vi "EOL CAN_Init CAL.vi"(5 "Parttype ref":refnum<vi>, 7 "Flash Size":i32, 8 "Glass?":bool=TRUE, 9 "Read Session in":refnum<k21>, 10 "DSC Write Session in":refnum<k21>, 11 "SA2 Operator":T1[](array[typedef]) {"Wert" format="%.0x"}) -> (1 "Error String Out":string, 2 "TxRx Data":string[][](array[string]), 3 "Response Good?":bool)   [LabVIEW 2014]
uses:
  Typedefs/Diagnose_SA2_Rechnenbefehl.ctl
  Typedefs/Diagnose_SA2_Operation_ENUM.ctl
  typedefs/parttype.ctl
  Typedefs/Select Session.ctl
  <vilib>/xnet/xnet.llb/XNET Frame CAN.ctl
  <vilib>/xnet/xnet.llb/XNET Frame Type CAN.ctl
panel:
  in  "Error String":string
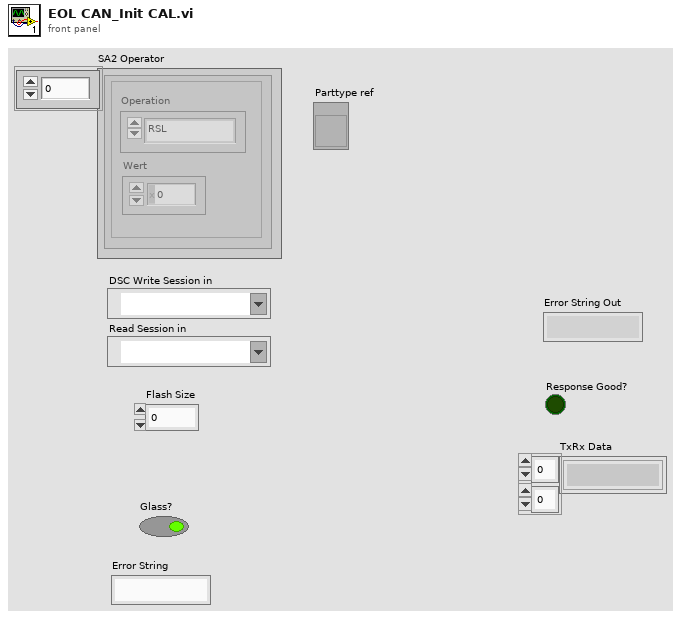
[diagram p1: front panel]
types:
  T1 = typedef "Diagnose_SA2_Rechnenbefehl.ctl" = cluster{"Operation":T2, "Wert":u32}
  T2 = typedef "Diagnose_SA2_Operation_ENUM.ctl" = enum16{"RSL", "RSR", "ADD", "SUB", "EOR", "Durchläufe", "NEXT", "BCC", "BRA", "Fertig"}
  T3 = cluster{"DSC Write Session in":refnum<k21>, "Read Session in":refnum<k21>, "Error String":string, "Response Good?":bool, "Glass?":bool, "TxRx Data":string[][], "SA2 Operator":T1[], "Flash Size":i32, "Parttype ref":refnum<vi>}
  T4 = typedef "Select Session.ctl" = enum16{"DefaultSession", "Development", "Extended", "EOL", "Programming"}
  T5 = typedef "XNET Frame CAN.ctl" = cluster{"timestamp":timestamp, "payload":u8[], "identifier":u32, "type":T6, "extended?":bool, "echo?":bool}
  T6 = typedef "XNET Frame Type CAN.ctl" = u8
  T7 = typedef "parttype.ctl" = enum16{"NMS", "B-SUV"}
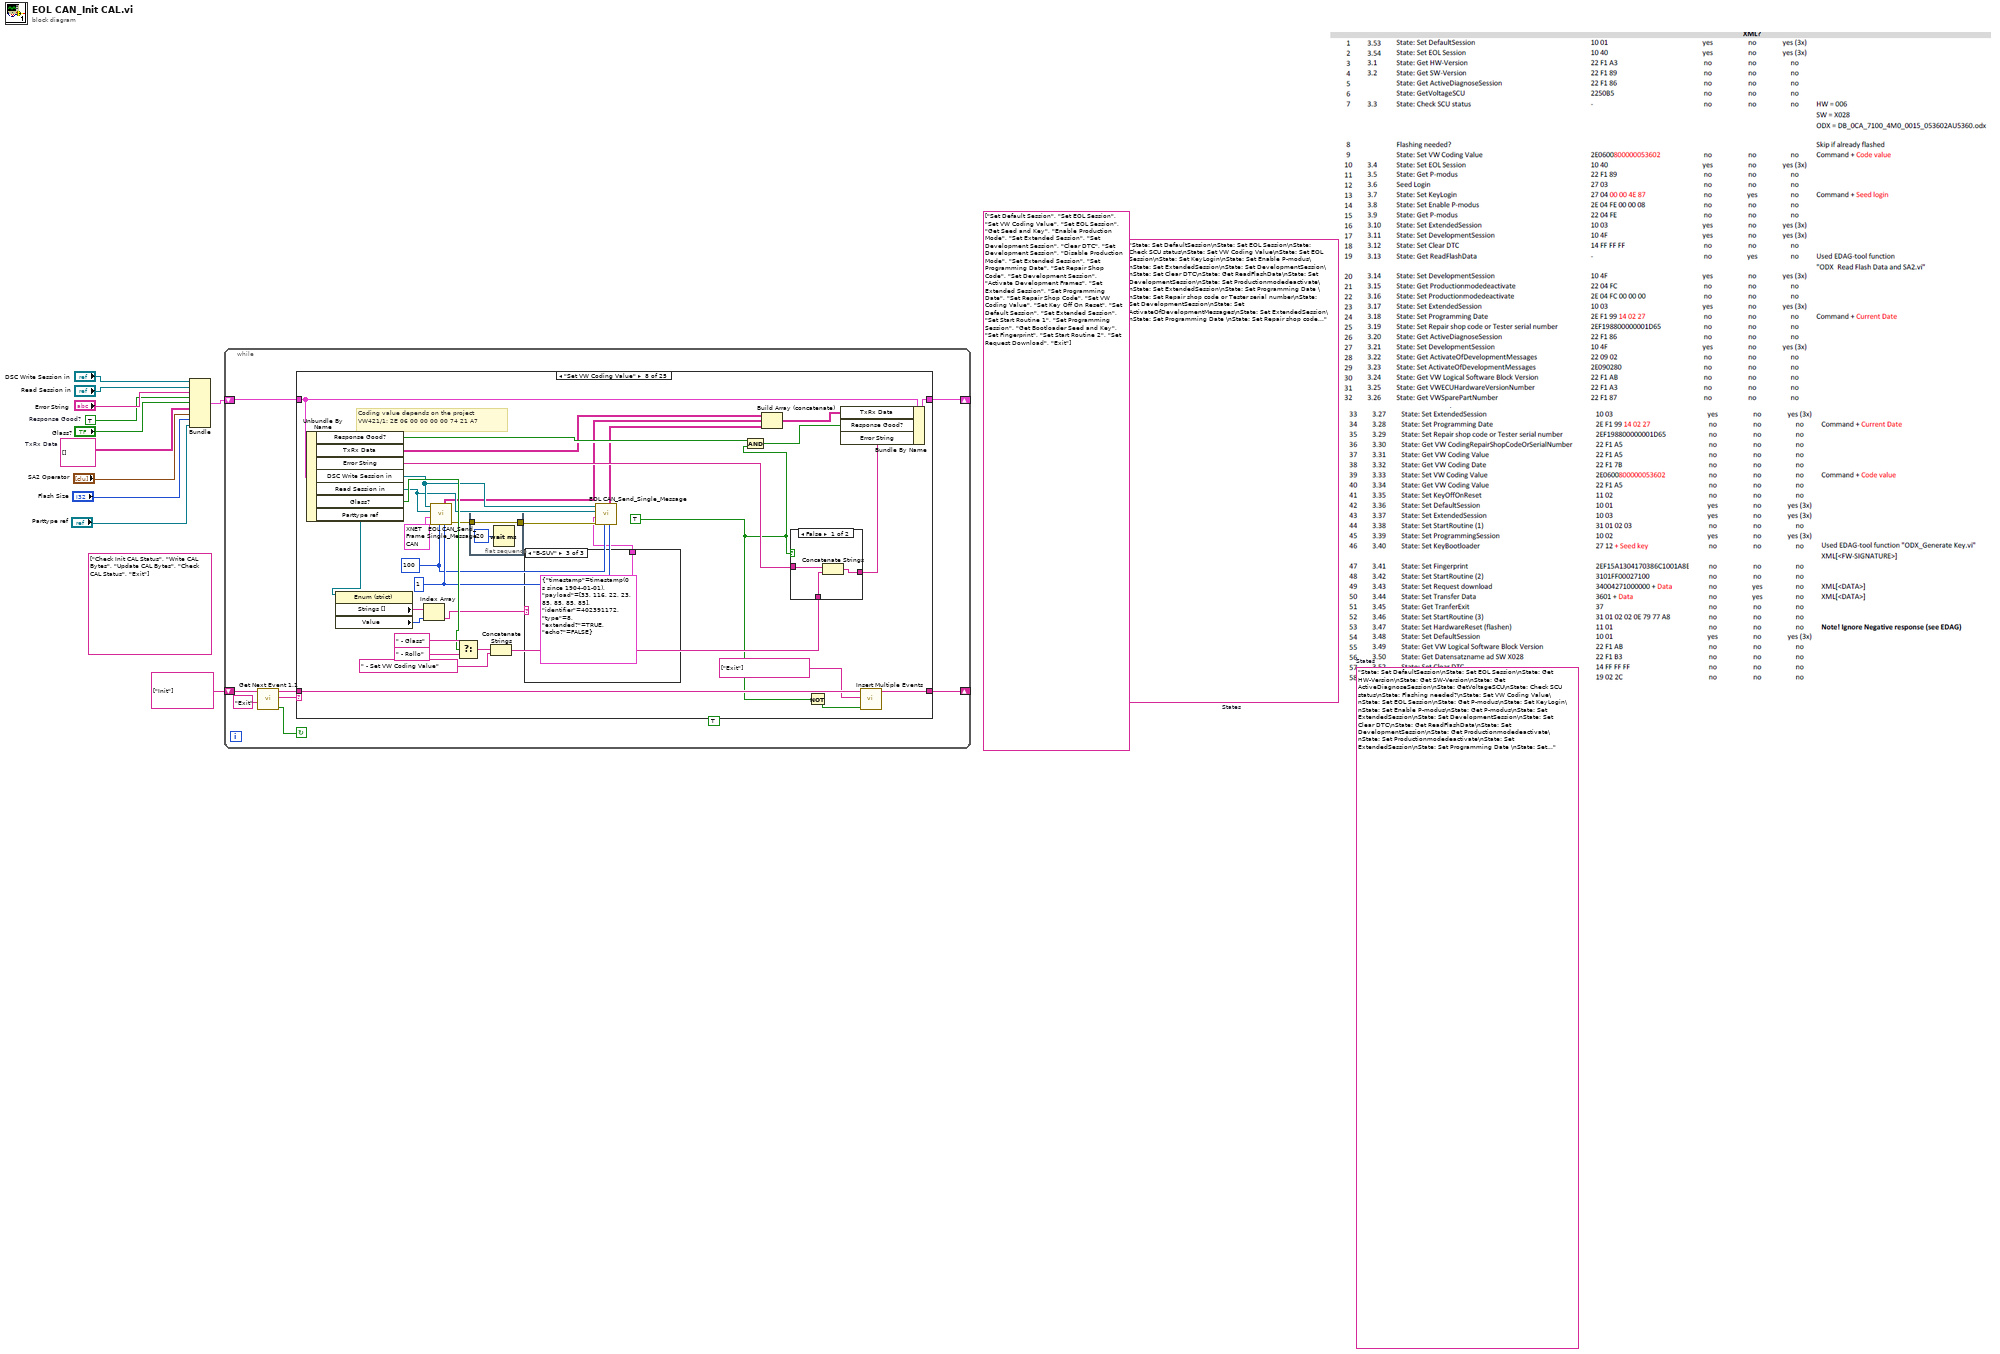
[diagram p0: block diagram]
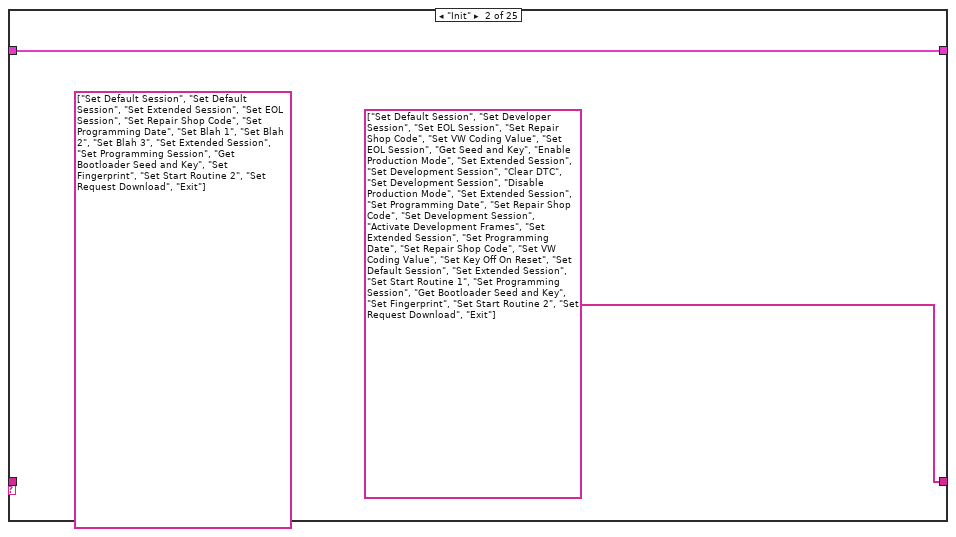
[diagram p3: hidden frame]
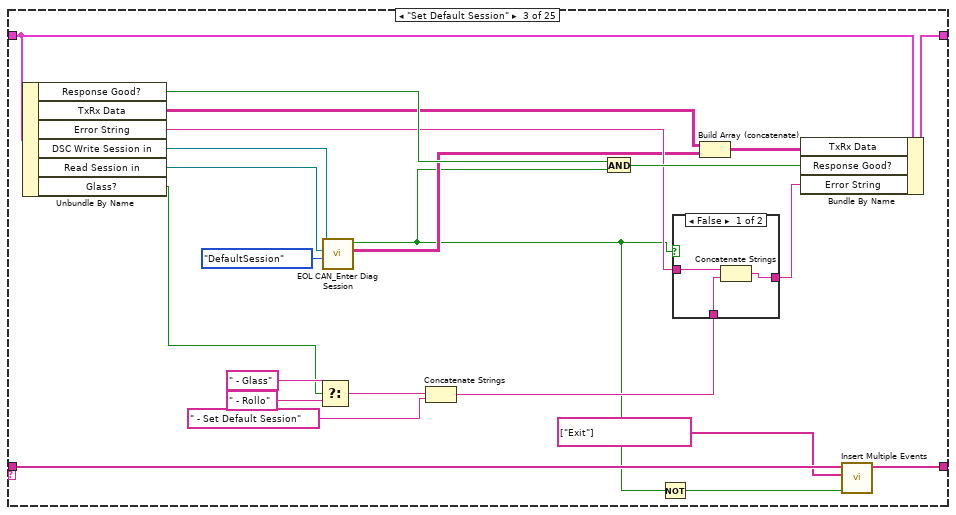
[diagram p4: hidden frame]
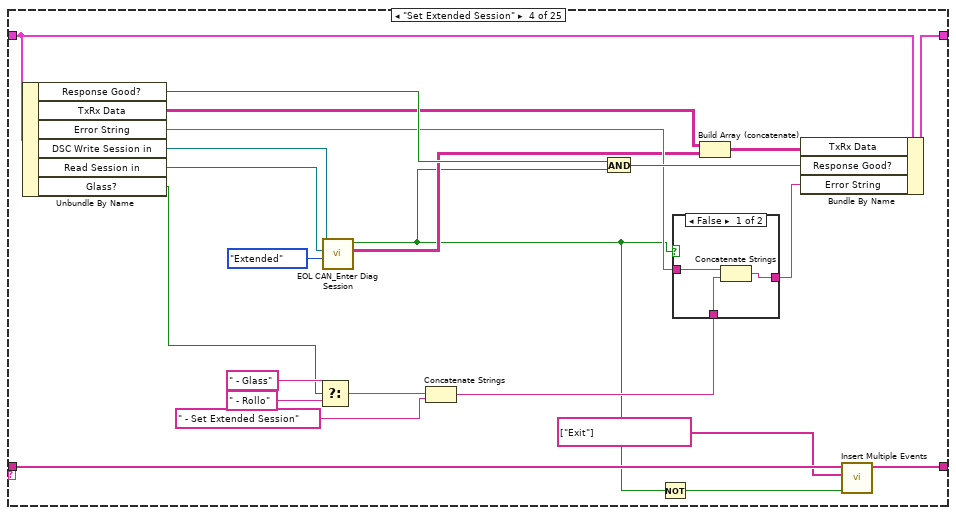
[diagram p6: hidden frame]
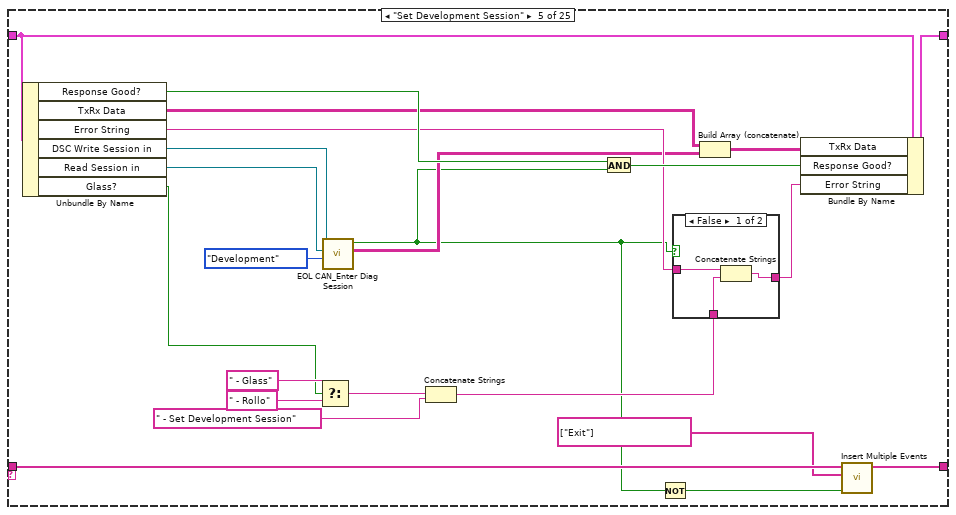
[diagram p8: hidden frame]
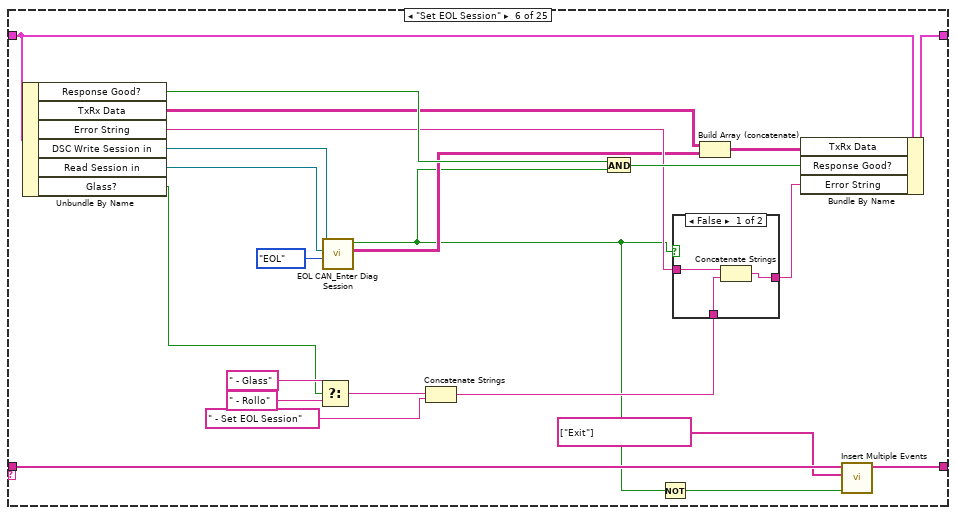
[diagram p10: hidden frame]
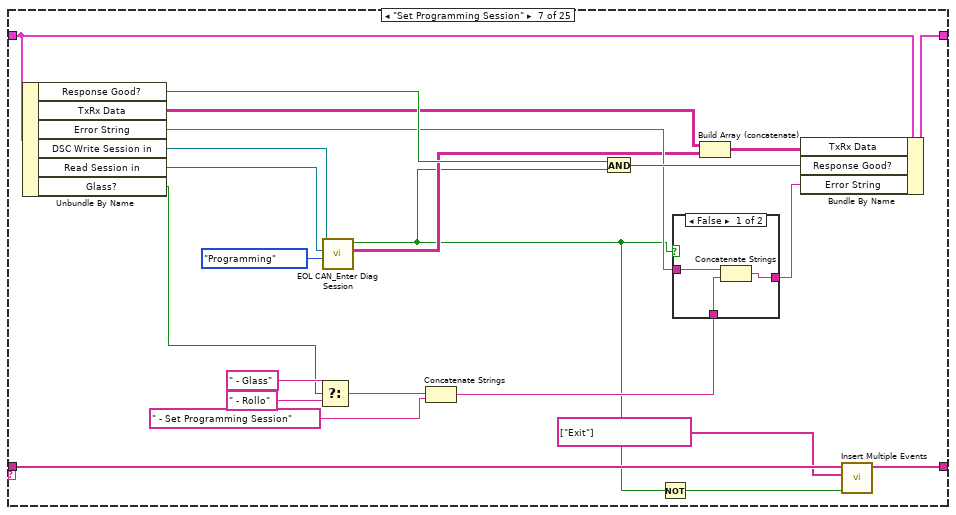
[diagram p12: hidden frame]
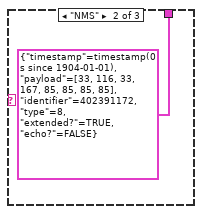
[diagram p15: hidden frame]
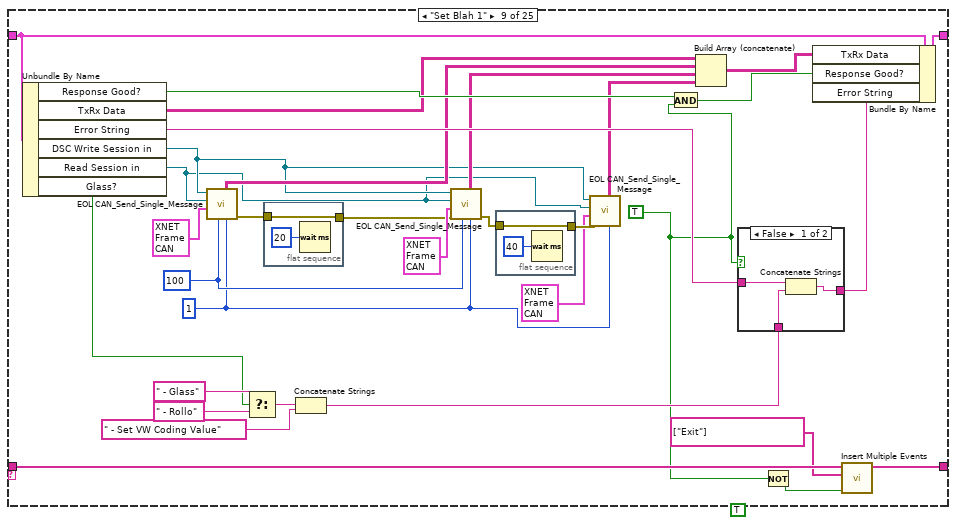
[diagram p17: hidden frame]
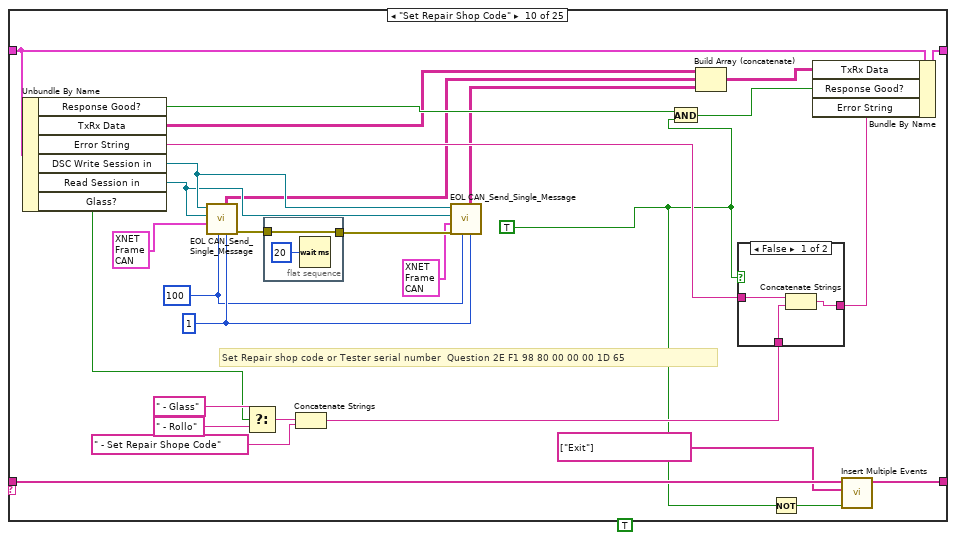
[diagram p19: hidden frame]
diagram:
  (unwired) "State: Set DefaultSession\nState: Set EOL Session\nState: Get HW-Version\nState: Get SW-Version\nState: Get ActiveDiagnoseSession\nState: GetVoltageSCU\nState: Check SCU status\nState: Flashing needed?\nState: Set VW Coding Value\nState: Set EOL Session\nState: Get P-modus\nState: Set KeyLogin\nState: Set Enable P-modus\nState: Get P-modus\nState: Set ExtendedSession\nState: Set DevelopmentSession\nState: Set Clear DTC\nState: Get ReadFlashData\nState: Set DevelopmentSession\nState: Get Productionmodedeactivate\nState: Set Productionmodedeactivate\nState: Set ExtendedSession\nState: Set Programming Date \nState: Set Repair shop code or Tester serial number\nState: Get ActiveDiagnoseSession \nState: Set DevelopmentSession\nState: Get ActivateOfDevelopmentMessages\nState: Set ActivateOfDevelopmentMessages\nState: Get VW Logical Software Block Version\nState: Get VWECUHardwareVersionNumber\nState: Get VWSparePartNumber\nState: Set ExtendedSession\nState: Set Programming Date \nState: Set Repair shop code or Tester serial number\nState: Get VW CodingRepairShopCodeOrSerialNumber\nState: Get VW Coding Value\nState: Get VW Coding Date\nState: Set VW Coding Value\nState: Get VW Coding Value\nState: Set KeyOffOnReset\nState: Set DefaultSession\nState: Set ExtendedSession\nState: Set StartRoutine (1)\nState: Set ProgrammingSession\nState: Set KeyBootloader\nState: Set Fingerprint\nState: Set StartRoutine (2)\nState: Set Request download\nState: Set Transfer Data\nState: Get TranferExit\nState: Set StartRoutine (3)\nState: Get ActiveDiagnoseSession \nState: Set HardwareReset (flashen)\nState: Set DefaultSession\nState: Get VW Logical Software Block Version\nState: Get Datensatzname ad SW X028\nState: Set Clear DTC\nState: Get DTC (TestFailed + Confirmed DTC)\nExit"  # States
  (unwired) "State: Set DefaultSession\nState: Set EOL Session\nState: Check SCU status\nState: Set VW Coding Value\nState: Set EOL Session\nState: Set KeyLogin\nState: Set Enable P-modus\nState: Set ExtendedSession\nState: Set DevelopmentSession\nState: Set Clear DTC\nState: Get ReadFlashData\nState: Set DevelopmentSession\nState: Set Productionmodedeactivate\nState: Set ExtendedSession\nState: Set Programming Date \nState: Set Repair shop code or Tester serial number\nState: Set DevelopmentSession\nState: Set ActivateOfDevelopmentMessages\nState: Set ExtendedSession\nState: Set Programming Date \nState: Set Repair shop code or Tester serial number\nState: Set VW Coding Value\nState: Set KeyOffOnReset\nState: Set DefaultSession\nState: Set ExtendedSession\nState: Set StartRoutine (1)\nState: Set ProgrammingSession\nState: Set KeyBootloader\nState: Set Fingerprint\nState: Set StartRoutine (2)\nState: Set Request download\nState: Set Transfer Data\nState: Get TranferExit\nState: Set StartRoutine (3)\nState: Set HardwareReset (flashen)\nState: Set DefaultSession\nState: Get Datensatzname ad SW X028\nState: Set Clear DTC\nState: Get DTC (TestFailed + Confirmed DTC)\nExit"  # States
  (unwired) string[] ["Set Default Session", "Set EOL Session", "Set VW Coding Value", "Set EOL Session", "Get Seed and Key", "Enable Production Mode", "Set Extended Session", "Set Development Session", "Clear DTC", "Set Development Session", "Disable Production Mode", "Set Extended Session", "Set Programming Date", "Set Repair Shop Code", "Set Development Session", "Activate Development Frames", "Set Extended Session", "Set Programming Date", "Set Repair Shop Code", "Set VW Coding Value", "Set Key Off On Reset", "Set Default Session", "Set Extended Session", "Set Start Routine 1", "Set Programming Session", "Get Bootloader Seed and Key", "Set Fingerprint", "Set Start Routine 2", "Set Request Download", "Exit"] ("event queue out")
  (unwired) string[] ["Check Init CAL Status", "Write CAL Bytes", "Update CAL Bytes", "Check CAL Status", "Exit"] ("event queue out")
  w6 = string[][] []  # TxRx Data
  w9 = TRUE  # Response Good?
  n1 = Bundle("DSC Write Session in"="DSC Write Session in", "Read Session in"="Read Session in", "Error String"="Error String", "Response Good?"=w9, "Glass?"="Glass?", "TxRx Data"=w6, "SA2 Operator"="SA2 Operator", "Flash Size"="Flash Size", "Parttype ref"="Parttype ref") -> (w8:T3)  [unwired: 1 in]
  n2 = while {
    shift-right: [w17] -> _
    shift-left: string[] ["Init"] ("event queue out") -> [w16]
    shift-right: [w14] -> _
    shift-left: w8 -> [w15]
    stop <- w19 continue-if-true
    n3 = call "Get Next Event 1.1.vi"("Exit Event"="Exit", "event queue in"=w16) -> ("Condition (Exit:F)"=w19:bool, "next event"=w12:string, "event queue out"=w18:string[])  [unwired: 6 in, 1 out]
    n4 = case shown="\"Set VW Coding Value\"" w12 {
      tunnel: w18 -> [w21 _ w34 w61 w88 w115 w142 w179 w220 w257 w298 w333 w361 w388 w414 w440 w477 w507 w538 w567 w594 w621 w648 w674 w695]
      tunnel: [w21 string[] ["Set Default Session", "Set Developer Session", "Set EOL Session", "Set Repair Shop Code", "Set VW Coding Value", "Set EOL Session", "Get Seed and Key", "Enable Production Mode", "Set Extended Session", "Set Development Session", "Clear DTC", "Set Development Session", "Disable Production Mode", "Set Extended Session", "Set Programming Date", "Set Repair Shop Code", "Set Development Session", "Activate Development Frames", "Set Extended Session", "Set Programming Date", "Set Repair Shop Code", "Set VW Coding Value", "Set Key Off On Reset", "Set Default Session", "Set Extended Session", "Set Start Routine 1", "Set Programming Session", "Get Bootloader Seed and Key", "Set Fingerprint", "Set Start Routine 2", "Set Request Download", "Exit"] ("event queue out") w35 w62 w89 w116 w143 w180 w221 w258 w299 w334 w362 w389 w415 w441 w478 w508 w539 w568 w595 w622 w649 w675 w695] -> w17
      tunnel: w15 -> [w20 w23 w45 w72 w99 w126 w153 w190 w231 w268 w309 w344 w372 w399 w425 w451 w488 w518 w549 w578 w605 w632 w659 w685 w694]
      tunnel: [w20 w23 w43 w70 w97 w124 w151 w188 w229 w266 w307 w342 w370 w397 w423 w449 w486 w516 w547 w576 w603 w630 w657 w683 w694] -> w14
      frame "Error", Default {
      }
      frame "Init" {
        (unwired) string[] ["Set Default Session", "Set Default Session", "Set Extended Session", "Set EOL Session", "Set Repair Shop Code", "Set Programming Date", "Set Blah 1", "Set Blah 2", "Set Blah 3", "Set Extended Session", "Set Programming Session", "Get Bootloader Seed and Key", "Set Fingerprint", "Set Start Routine 2", "Set Request Download", "Exit"] ("event queue out")
        # "Inalfa Sequences"
        # "Conti-Sequences"
      }
      frame "Set Default Session" {
        n5 = Unbundle By Name(w45) -> ("Response Good?"=w46:bool, "TxRx Data"=w32:string[][], "Error String"=w42:string, "DSC Write Session in"=w29:refnum<k21>, "Read Session in"=w28:refnum<k21>, "Glass?"=w26:bool)
        n6 = Select(t=" - Glass" ("Error Description"), s=w26, f=" - Rollo" ("Error Description")) -> (s? t:f=w40:string)
        n7 = call "EOL CAN_Enter Diag Session.vi"("Session"=Select_Session."DefaultSession", "Read Session in"=w28, "Write Session in"=w29) -> ("TxRx Data"=w30:string[][], "Response Good?"=w25:bool)  [unwired: 6 in, 1 out]
        n8 = Concatenate Strings(w40, " - Set Default Session" ("Error Description")) -> (w36:string)
        n9 = And(x=w46, y=w25) -> (x .and. y?=w44:bool)
        n10 = Not(x=w25) -> (.not. x?=w24:bool)
        n11 = case shown="False" w25 {
          tunnel: w42 -> [w48 w50]
          tunnel: [w49 w50] -> w41
          tunnel: w36 -> [w47 _]
          frame False {
            n12 = Concatenate Strings(w48, w47) -> (w49:string)
          }
          frame True {
          }
        }
        n13 = Build Array (concatenate)(w32, w30) -> (w31:string[][])
        n14 = Bundle By Name(cluster=w45, "TxRx Data"=w31, "Response Good?"=w44, "Error String"=w41) -> (w43:T3)
        n15 = call "Insert Multiple Events.vi"("Insert all? (T)"=w24, "Events to Insert"=string[] ["Exit"], "Event queue in"=w34) -> ("Event queue out"=w35:string[])  [unwired: 4 in]
      }
      frame "Set Extended Session" {
        n16 = Unbundle By Name(w72) -> ("Response Good?"=w73:bool, "TxRx Data"=w59:string[][], "Error String"=w69:string, "DSC Write Session in"=w56:refnum<k21>, "Read Session in"=w55:refnum<k21>, "Glass?"=w53:bool)
        n17 = Select(t=" - Glass" ("Error Description"), s=w53, f=" - Rollo" ("Error Description")) -> (s? t:f=w67:string)
        n18 = call "EOL CAN_Enter Diag Session.vi"("Session"=Select_Session."Extended", "Read Session in"=w55, "Write Session in"=w56) -> ("TxRx Data"=w57:string[][], "Response Good?"=w52:bool)  [unwired: 6 in, 1 out]
        n19 = Concatenate Strings(w67, " - Set Extended Session" ("Error Description")) -> (w63:string)
        n20 = And(x=w73, y=w52) -> (x .and. y?=w71:bool)
        n21 = Not(x=w52) -> (.not. x?=w51:bool)
        n22 = case shown="False" w52 {
          tunnel: w69 -> [w75 w77]
          tunnel: [w76 w77] -> w68
          tunnel: w63 -> [w74 _]
          frame False {
            n23 = Concatenate Strings(w75, w74) -> (w76:string)
          }
          frame True {
          }
        }
        n24 = Build Array (concatenate)(w59, w57) -> (w58:string[][])
        n25 = Bundle By Name(cluster=w72, "TxRx Data"=w58, "Response Good?"=w71, "Error String"=w68) -> (w70:T3)
        n26 = call "Insert Multiple Events.vi"("Insert all? (T)"=w51, "Events to Insert"=string[] ["Exit"], "Event queue in"=w61) -> ("Event queue out"=w62:string[])  [unwired: 4 in]
      }
      frame "Set Development Session" {
        n27 = Unbundle By Name(w99) -> ("Response Good?"=w100:bool, "TxRx Data"=w86:string[][], "Error String"=w96:string, "DSC Write Session in"=w83:refnum<k21>, "Read Session in"=w82:refnum<k21>, "Glass?"=w80:bool)
        n28 = Select(t=" - Glass" ("Error Description"), s=w80, f=" - Rollo" ("Error Description")) -> (s? t:f=w94:string)
        n29 = call "EOL CAN_Enter Diag Session.vi"("Session"=Select_Session."Development", "Read Session in"=w82, "Write Session in"=w83) -> ("TxRx Data"=w84:string[][], "Response Good?"=w79:bool)  [unwired: 6 in, 1 out]
        n30 = Concatenate Strings(w94, " - Set Development Session" ("Error Description")) -> (w90:string)
        n31 = And(x=w100, y=w79) -> (x .and. y?=w98:bool)
        n32 = Not(x=w79) -> (.not. x?=w78:bool)
        n33 = case shown="False" w79 {
          tunnel: w96 -> [w102 w104]
          tunnel: [w103 w104] -> w95
          tunnel: w90 -> [w101 _]
          frame False {
            n34 = Concatenate Strings(w102, w101) -> (w103:string)
          }
          frame True {
          }
        }
        n35 = Build Array (concatenate)(w86, w84) -> (w85:string[][])
        n36 = Bundle By Name(cluster=w99, "TxRx Data"=w85, "Response Good?"=w98, "Error String"=w95) -> (w97:T3)
        n37 = call "Insert Multiple Events.vi"("Insert all? (T)"=w78, "Events to Insert"=string[] ["Exit"], "Event queue in"=w88) -> ("Event queue out"=w89:string[])  [unwired: 4 in]
      }
      frame "Set EOL Session" {
        n38 = Unbundle By Name(w126) -> ("Response Good?"=w127:bool, "TxRx Data"=w113:string[][], "Error String"=w123:string, "DSC Write Session in"=w110:refnum<k21>, "Read Session in"=w109:refnum<k21>, "Glass?"=w107:bool)
        n39 = Select(t=" - Glass" ("Error Description"), s=w107, f=" - Rollo" ("Error Description")) -> (s? t:f=w121:string)
        n40 = call "EOL CAN_Enter Diag Session.vi"("Session"=Select_Session."EOL", "Read Session in"=w109, "Write Session in"=w110) -> ("TxRx Data"=w111:string[][], "Response Good?"=w106:bool)  [unwired: 6 in, 1 out]
        n41 = Concatenate Strings(w121, " - Set EOL Session" ("Error Description")) -> (w117:string)
        n42 = And(x=w127, y=w106) -> (x .and. y?=w125:bool)
        n43 = Not(x=w106) -> (.not. x?=w105:bool)
        n44 = case shown="False" w106 {
          tunnel: w123 -> [w129 w131]
          tunnel: [w130 w131] -> w122
          tunnel: w117 -> [w128 _]
          frame False {
            n45 = Concatenate Strings(w129, w128) -> (w130:string)
          }
          frame True {
          }
        }
        n46 = Build Array (concatenate)(w113, w111) -> (w112:string[][])
        n47 = Bundle By Name(cluster=w126, "TxRx Data"=w112, "Response Good?"=w125, "Error String"=w122) -> (w124:T3)
        n48 = call "Insert Multiple Events.vi"("Insert all? (T)"=w105, "Events to Insert"=string[] ["Exit"], "Event queue in"=w115) -> ("Event queue out"=w116:string[])  [unwired: 4 in]
      }
      frame "Set Programming Session" {
        n49 = Unbundle By Name(w153) -> ("Response Good?"=w154:bool, "TxRx Data"=w140:string[][], "Error String"=w150:string, "DSC Write Session in"=w137:refnum<k21>, "Read Session in"=w136:refnum<k21>, "Glass?"=w134:bool)
        n50 = Select(t=" - Glass" ("Error Description"), s=w134, f=" - Rollo" ("Error Description")) -> (s? t:f=w148:string)
        n51 = call "EOL CAN_Enter Diag Session.vi"("Session"=Select_Session."Programming", "Read Session in"=w136, "Write Session in"=w137) -> ("TxRx Data"=w138:string[][], "Response Good?"=w133:bool)  [unwired: 6 in, 1 out]
        n52 = Concatenate Strings(w148, " - Set Programming Session" ("Error Description")) -> (w144:string)
        n53 = And(x=w154, y=w133) -> (x .and. y?=w152:bool)
        n54 = Not(x=w133) -> (.not. x?=w132:bool)
        n55 = case shown="False" w133 {
          tunnel: w150 -> [w156 w158]
          tunnel: [w157 w158] -> w149
          tunnel: w144 -> [w155 _]
          frame False {
            n56 = Concatenate Strings(w156, w155) -> (w157:string)
          }
          frame True {
          }
        }
        n57 = Build Array (concatenate)(w140, w138) -> (w139:string[][])
        n58 = Bundle By Name(cluster=w153, "TxRx Data"=w139, "Response Good?"=w152, "Error String"=w149) -> (w151:T3)
        n59 = call "Insert Multiple Events.vi"("Insert all? (T)"=w132, "Events to Insert"=string[] ["Exit"], "Event queue in"=w142) -> ("Event queue out"=w143:string[])  [unwired: 4 in]
      }
      frame "Set VW Coding Value" {
        w164 = TRUE ("Response Good?")
        (unwired) TRUE ("Insert all? (T)")
        w171 = 1 ("Retries")
        w170 = u32 100 ("Msg Wait Time")
        # "Coding value depends on the project\nVW421/1: 2E 06 00 00 00 00 74 21 A7"
        n60 = Unbundle By Name(w190) -> ("Response Good?"=w191:bool, "TxRx Data"=w177:string[][], "Error String"=w187:string, "DSC Write Session in"=w173:refnum<k21>, "Read Session in"=w172:refnum<k21>, "Glass?"=w175:bool, "Parttype ref"=w160:refnum<vi>)
        n61 = property class="Enum (strict)"(reference=w160) -> ("Strings []"=w161:string[], "Value"=w162:T7)  [unwired: 1 in, 2 out]
        n62 = Index Array(array=w161, index=w162) -> (element=w159:string)
        n63 = call "EOL CAN_Send_Single_Message.vi"("Retries"=w171, "Msg Wait Time"=w170, "Tx CAN frame"=T5 {"timestamp"=timestamp(0 s since 1904-01-01), "payload"=[16, 9, 46, 6, 0, 0, 0, 0], "identifier"=402391172, "type"=8, "extended?"=TRUE, "echo?"=FALSE}, "Read Session in"=w172, "Write Session in"=w173) -> ("Error out"=w167:errorcluster, "TxRx Data"=w169:string[][])  [unwired: 2 in, 3 out]
        n64 = Select(t=" - Glass" ("Error Description"), s=w175, f=" - Rollo" ("Error Description")) -> (s? t:f=w185:string)
        n65 = flat-sequence {
          tunnel: w167 -> [w195]
          tunnel: [w195] -> w166
          frame #0 {
            n66 = Wait (ms)(milliseconds to wait=u32 20) -> ()  [unwired: 1 out]
          }
        }
        n67 = Concatenate Strings(w185, " - Set VW Coding Value" ("Error Description")) -> (w181:string)
        n68 = case shown="\"B-SUV\"" w159 {
          tunnel: [_ T5 {"timestamp"=timestamp(0 s since 1904-01-01), "payload"=[33, 116, 33, 167, 85, 85, 85, 85], "identifier"=402391172, "type"=8, "extended?"=TRUE, "echo?"=FALSE} ("Tx CAN frame") T5 {"timestamp"=timestamp(0 s since 1904-01-01), "payload"=[33, 116, 22, 23, 85, 85, 85, 85], "identifier"=402391172, "type"=8, "extended?"=TRUE, "echo?"=FALSE} ("Tx CAN frame")] -> w163
          frame "NaN", Default {
          }
          frame "NMS" {
          }
          frame "B-SUV" {
          }
        }
        n69 = call "EOL CAN_Send_Single_Message.vi"("Retries"=w171, "Msg Wait Time"=w170, "Error in"=w166, "Tx CAN frame"=w163, "Read Session in"=w172, "Write Session in"=w173) -> ("TxRx Data"=w168:string[][])  [unwired: 1 in, 4 out]
        n70 = And(x=w191, y=w164) -> (x .and. y?=w189:bool)
        n71 = Build Array (concatenate)(w177, w169, w168) -> (w176:string[][])
        n72 = case shown="False" w164 {
          tunnel: w187 -> [w197 w199]
          tunnel: [w198 w199] -> w186
          tunnel: w181 -> [w196 _]
          frame False {
            n73 = Concatenate Strings(w197, w196) -> (w198:string)
          }
          frame True {
          }
        }
        n74 = Not(x=w164) -> (.not. x?=w165:bool)
        n75 = Bundle By Name(cluster=w190, "TxRx Data"=w176, "Response Good?"=w189, "Error String"=w186) -> (w188:T3)
        n76 = call "Insert Multiple Events.vi"("Insert all? (T)"=w165, "Events to Insert"=string[] ["Exit"], "Event queue in"=w179) -> ("Event queue out"=w180:string[])  [unwired: 4 in]
      }
      frame "Set Blah 1" {
        w207 = TRUE ("Response Good?")
        (unwired) TRUE ("Insert all? (T)")
        w200 = 1 ("Retries")
        w213 = u32 100 ("Msg Wait Time")
        n77 = Unbundle By Name(w231) -> ("Response Good?"=w232:bool, "TxRx Data"=w218:string[][], "Error String"=w228:string, "DSC Write Session in"=w204:refnum<k21>, "Read Session in"=w203:refnum<k21>, "Glass?"=w216:bool)
        n78 = call "EOL CAN_Send_Single_Message.vi"("Retries"=w200, "Msg Wait Time"=w213, "Tx CAN frame"=T5 {"timestamp"=timestamp(0 s since 1904-01-01), "payload"=[16, 14, 46, 241, 160, 67, 111, 110], "identifier"=402391172, "type"=8, "extended?"=TRUE, "echo?"=FALSE}, "Read Session in"=w203, "Write Session in"=w204) -> ("Error out"=w210:errorcluster, "TxRx Data"=w212:string[][])  [unwired: 2 in, 3 out]
        n79 = Select(t=" - Glass" ("Error Description"), s=w216, f=" - Rollo" ("Error Description")) -> (s? t:f=w226:string)
        n80 = flat-sequence {
          tunnel: w210 -> [w236]
          tunnel: [w236] -> w209
          frame #0 {
            n81 = Wait (ms)(milliseconds to wait=u32 20) -> ()  [unwired: 1 out]
          }
        }
        n82 = Concatenate Strings(w226, " - Set VW Coding Value" ("Error Description")) -> (w222:string)
        n83 = call "EOL CAN_Send_Single_Message.vi"("Retries"=w200, "Msg Wait Time"=w213, "Error in"=w209, "Tx CAN frame"=T5 {"timestamp"=timestamp(0 s since 1904-01-01), "payload"=[33, 116, 105, 110, 101, 110, 116, 97], "identifier"=402391172, "type"=8, "extended?"=TRUE, "echo?"=FALSE}, "Read Session in"=w203, "Write Session in"=w204) -> ("Error out"=w206:errorcluster, "TxRx Data"=w211:string[][])  [unwired: 1 in, 3 out]
        n84 = flat-sequence {
          tunnel: w206 -> [w234]
          tunnel: [w234] -> w205
          frame #0 {
            n85 = Wait (ms)(milliseconds to wait=u32 40) -> ()  [unwired: 1 out]
          }
        }
        n86 = call "EOL CAN_Send_Single_Message.vi"("Retries"=w200, "Error in"=w205, "Tx CAN frame"=T5 {"timestamp"=timestamp(0 s since 1904-01-01), "payload"=[34, 108, 85, 85, 85, 85, 85, 85], "identifier"=402391172, "type"=8, "extended?"=TRUE, "echo?"=FALSE}, "Read Session in"=w203, "Write Session in"=w204) -> ("TxRx Data"=w201:string[][])  [unwired: 2 in, 4 out]
        n87 = And(x=w232, y=w207) -> (x .and. y?=w230:bool)
        n88 = Build Array (concatenate)(w218, w212, w211, w201) -> (w217:string[][])
        n89 = case shown="False" w207 {
          tunnel: w228 -> [w238 w240]
          tunnel: [w239 w240] -> w227
          tunnel: w222 -> [w237 _]
          frame False {
            n90 = Concatenate Strings(w238, w237) -> (w239:string)
          }
          frame True {
          }
        }
        n91 = Not(x=w207) -> (.not. x?=w208:bool)
        n92 = Bundle By Name(cluster=w231, "TxRx Data"=w217, "Response Good?"=w230, "Error String"=w227) -> (w229:T3)
        n93 = call "Insert Multiple Events.vi"("Insert all? (T)"=w208, "Events to Insert"=string[] ["Exit"], "Event queue in"=w220) -> ("Event queue out"=w221:string[])  [unwired: 4 in]
      }
      frame "Set Repair Shop Code" {
        w243 = TRUE ("Response Good?")
        (unwired) TRUE ("Insert all? (T)")
        w250 = 1 ("Retries")
        w249 = u32 100 ("Msg Wait Time")
        # "Set Repair shop code or Tester serial number \tQuestion\t2E F1 98 80 00 00 00 1D 65"
        n94 = Unbundle By Name(w268) -> ("Response Good?"=w269:bool, "TxRx Data"=w255:string[][], "Error String"=w265:string, "DSC Write Session in"=w252:refnum<k21>, "Read Session in"=w251:refnum<k21>, "Glass?"=w253:bool)
        n95 = call "EOL CAN_Send_Single_Message.vi"("Retries"=w250, "Msg Wait Time"=w249, "Tx CAN frame"=T5 {"timestamp"=timestamp(0 s since 1904-01-01), "payload"=[16, 9, 46, 241, 152, 128, 0, 0], "identifier"=402391172, "type"=8, "extended?"=TRUE, "echo?"=FALSE}, "Read Session in"=w251, "Write Session in"=w252) -> ("Error out"=w246:errorcluster, "TxRx Data"=w248:string[][])  [unwired: 2 in, 3 out]
        n96 = Select(t=" - Glass" ("Error Description"), s=w253, f=" - Rollo" ("Error Description")) -> (s? t:f=w263:string)
        n97 = flat-sequence {
          tunnel: w246 -> [w271]
          tunnel: [w271] -> w245
          frame #0 {
            n98 = Wait (ms)(milliseconds to wait=u32 20) -> ()  [unwired: 1 out]
          }
        }
        n99 = Concatenate Strings(w263, " - Set Repair Shope Code" ("Error Description")) -> (w259:string)
        n100 = call "EOL CAN_Send_Single_Message.vi"("Retries"=w250, "Msg Wait Time"=w249, "Error in"=w245, "Tx CAN frame"=T5 {"timestamp"=timestamp(0 s since 1904-01-01), "payload"=[33, 0, 29, 101, 85, 85, 85, 85], "identifier"=402391172, "type"=8, "extended?"=TRUE, "echo?"=FALSE}, "Read Session in"=w251, "Write Session in"=w252) -> ("TxRx Data"=w247:string[][])  [unwired: 1 in, 4 out]
        n101 = And(x=w269, y=w243) -> (x .and. y?=w267:bool)
        n102 = Build Array (concatenate)(w255, w248, w247) -> (w254:string[][])
        n103 = case shown="False" w243 {
          tunnel: w265 -> [w273 w275]
          tunnel: [w274 w275] -> w264
          tunnel: w259 -> [w272 _]
          frame False {
            n104 = Concatenate Strings(w273, w272) -> (w274:string)
          }
          frame True {
          }
        }
        n105 = Not(x=w243) -> (.not. x?=w244:bool)
        n106 = Bundle By Name(cluster=w268, "TxRx Data"=w254, "Response Good?"=w267, "Error String"=w264) -> (w266:T3)
        n107 = call "Insert Multiple Events.vi"("Insert all? (T)"=w244, "Events to Insert"=string[] ["Exit"], "Event queue in"=w257) -> ("Event queue out"=w258:string[])  [unwired: 4 in]
      }
      frame "Set Request Download" {
        w284 = TRUE
        (unwired) TRUE ("Insert all? (T)")
        w290 = u32 100 ("Msg Wait Time")
        n108 = Unbundle By Name(w309) -> ("Response Good?"=w310:bool, "TxRx Data"=w296:string[][], "Error String"=w306:string, "DSC Write Session in"=w293:refnum<k21>, "Read Session in"=w292:refnum<k21>, "Flash Size"=w281:i32, "Glass?"=w294:bool)
        n109 = call "create request byte.vi"("x"=w281) -> ("output array 2"=w277:u8[], "output array"=w280:u8[])  [unwired: 9 in]
        n110 = Bundle By Name(cluster=T5 {"timestamp"=timestamp(0 s since 1904-01-01), "payload"=[16, 9, 52, 0, 66, 0, 0, 0], "identifier"=402391172, "type"=8, "extended?"=TRUE, "echo?"=FALSE} ("Tx CAN frame"), "payload"=w280) -> (w282:T5)
        n111 = Select(t=" - Glass" ("Error Description"), s=w294, f=" - Rollo" ("Error Description")) -> (s? t:f=w304:string)
        n112 = call "EOL CAN_Send_Single_Message.vi"("Retries"=1, "Msg Wait Time"=w290, "Tx CAN frame"=w282, "Read Session in"=w292, "Write Session in"=w293) -> ("Error out"=w287:errorcluster, "TxRx Data"=w289:string[][])  [unwired: 2 in, 3 out]
        n113 = Concatenate Strings(w304, " - Set Repair Shope Code" ("Error Description")) -> (w300:string)
        n114 = flat-sequence {
          tunnel: w287 -> [w312]
          tunnel: [w312] -> w286
          frame #0 {
            n115 = Wait (ms)(milliseconds to wait=u32 10) -> ()  [unwired: 1 out]
          }
        }
        n116 = Bundle By Name(cluster=T5 {"timestamp"=timestamp(0 s since 1904-01-01), "payload"=[33, 0, 0, 0, 0, 85, 85, 85], "identifier"=402391172, "type"=8, "extended?"=TRUE, "echo?"=FALSE} ("Tx CAN frame"), "payload"=w277) -> (w278:T5)
        n117 = call "EOL CAN_Send_Single_Message.vi"("Retries"=1, "Msg Wait Time"=w290, "Error in"=w286, "Tx CAN frame"=w278, "Read Session in"=w292, "Write Session in"=w293) -> ("TxRx Data"=w288:string[][])  [unwired: 1 in, 4 out]
        n118 = And(x=w310, y=w284) -> (x .and. y?=w308:bool)
        n119 = Build Array (concatenate)(w296, w289, w288) -> (w295:string[][])
        n120 = case shown="False" w284 {
          tunnel: w306 -> [w314 w316]
          tunnel: [w315 w316] -> w305
          tunnel: w300 -> [w313 _]
          frame False {
            n121 = Concatenate Strings(w314, w313) -> (w315:string)
          }
          frame True {
          }
        }
        n122 = Not(x=w284) -> (.not. x?=w285:bool)
        n123 = Bundle By Name(cluster=w309, "TxRx Data"=w295, "Response Good?"=w308, "Error String"=w305) -> (w307:T3)
        n124 = call "Insert Multiple Events.vi"("Insert all? (T)"=w285, "Events to Insert"=string[] ["Exit"], "Event queue in"=w298) -> ("Event queue out"=w299:string[])  [unwired: 4 in]
      }
      frame "Set Fingerprint" {
        (unwired) T5 {"timestamp"=timestamp(0 s since 1904-01-01), "payload"=[16, 12, 46, 241, 90, 23, 4, 39], "identifier"=402391172, "type"=8, "extended?"=TRUE, "echo?"=FALSE} ("Tx CAN frame")
        (unwired) T5 {"timestamp"=timestamp(0 s since 1904-01-01), "payload"=[33, 60, 85, 68, 98, 103, 62, 85], "identifier"=402391172, "type"=8, "extended?"=TRUE, "echo?"=FALSE} ("Tx CAN frame")
        w318 = TRUE
        (unwired) TRUE ("Insert all? (T)")
        w326 = 1 ("Retries")
        w325 = u32 100 ("Msg Wait Time")
        # "Set Fingerprint \tQuestion\t2E F1 5A 13 04 17 03 86 C1 00 1A 8B"
        n125 = Unbundle By Name(w344) -> ("Response Good?"=w345:bool, "TxRx Data"=w331:string[][], "Error String"=w341:string, "DSC Write Session in"=w328:refnum<k21>, "Read Session in"=w327:refnum<k21>, "Glass?"=w329:bool)
        n126 = Select(t=" - Glass" ("Error Description"), s=w329, f=" - Rollo" ("Error Description")) -> (s? t:f=w339:string)
        n127 = call "EOL CAN_Send_Single_Message.vi"("Retries"=w326, "Msg Wait Time"=w325, "Tx CAN frame"=T5 {"timestamp"=timestamp(0 s since 1904-01-01), "payload"=[16, 12, 46, 241, 90, 19, 4, 23], "identifier"=402391172, "type"=8, "extended?"=TRUE, "echo?"=FALSE}, "Read Session in"=w327, "Write Session in"=w328) -> ("Error out"=w322:errorcluster, "TxRx Data"=w324:string[][])  [unwired: 2 in, 3 out]
        n128 = Concatenate Strings(w339, " - Set Fingerprint" ("Error Description")) -> (w335:string)
        n129 = flat-sequence {
          tunnel: w322 -> [w347]
          tunnel: [w347] -> w321
          frame #0 {
            n130 = Wait (ms)(milliseconds to wait=u32 20) -> ()  [unwired: 1 out]
          }
        }
        n131 = call "EOL CAN_Send_Single_Message.vi"("Retries"=w326, "Msg Wait Time"=w325, "Error in"=w321, "Tx CAN frame"=T5 {"timestamp"=timestamp(0 s since 1904-01-01), "payload"=[33, 3, 134, 193, 0, 26, 139, 85], "identifier"=402391172, "type"=8, "extended?"=TRUE, "echo?"=FALSE}, "Read Session in"=w327, "Write Session in"=w328) -> ("TxRx Data"=w323:string[][])  [unwired: 1 in, 4 out]
        n132 = And(x=w345, y=w318) -> (x .and. y?=w343:bool)
        n133 = Build Array (concatenate)(w331, w324, w323) -> (w330:string[][])
        n134 = case shown="False" w318 {
          tunnel: w341 -> [w349 w351]
          tunnel: [w350 w351] -> w340
          tunnel: w335 -> [w348 _]
          frame False {
            n135 = Concatenate Strings(w349, w348) -> (w350:string)
          }
          frame True {
          }
        }
        n136 = Not(x=w318) -> (.not. x?=w319:bool)
        n137 = Bundle By Name(cluster=w344, "TxRx Data"=w330, "Response Good?"=w343, "Error String"=w340) -> (w342:T3)
        n138 = call "Insert Multiple Events.vi"("Insert all? (T)"=w319, "Events to Insert"=string[] ["Exit"], "Event queue in"=w333) -> ("Event queue out"=w334:string[])  [unwired: 4 in]
      }
      frame "Get Login Seed and Key" {
        n139 = Unbundle By Name(w372) -> ("Response Good?"=w373:bool, "TxRx Data"=w359:string[][], "Error String"=w369:string, "DSC Write Session in"=w355:refnum<k21>, "Read Session in"=w354:refnum<k21>, "Glass?"=w357:bool)
        n140 = Select(t=" - Glass" ("Error Description"), s=w357, f=" - Rollo" ("Error Description")) -> (s? t:f=w367:string)
        n141 = Concatenate Strings(w367, " - Get Login Seed and Key" ("Error Description")) -> (w363:string)
        n142 = call "EOL CAN_Get Seed and Key.vi"("Read Session in"=w354, "Write Session in"=w355) -> ("Response Good?"=w352:bool, "TxRx Data"=w353:string[][])  [unwired: 7 in, 1 out]
        n143 = And(x=w373, y=w352) -> (x .and. y?=w371:bool)
        n144 = Build Array (concatenate)(w359, w353) -> (w358:string[][])
        n145 = Not(x=w352) -> (.not. x?=w356:bool)
        n146 = case shown="False" w352 {
          tunnel: w369 -> [w375 w377]
          tunnel: [w376 w377] -> w368
          tunnel: w363 -> [w374 _]
          frame False {
            n147 = Concatenate Strings(w375, w374) -> (w376:string)
          }
          frame True {
          }
        }
        n148 = Bundle By Name(cluster=w372, "TxRx Data"=w358, "Response Good?"=w371, "Error String"=w368) -> (w370:T3)
        n149 = call "Insert Multiple Events.vi"("Insert all? (T)"=w356, "Events to Insert"=string[] ["Exit"], "Event queue in"=w361) -> ("Event queue out"=w362:string[])  [unwired: 4 in]
      }
      frame "Get Bootloader Seed and Key" {
        n150 = Unbundle By Name(w399) -> ("Response Good?"=w400:bool, "TxRx Data"=w386:string[][], "Error String"=w396:string, "DSC Write Session in"=w381:refnum<k21>, "Read Session in"=w380:refnum<k21>, "SA2 Operator"=w382:T1[], "Glass?"=w384:bool)
        n151 = Select(t=" - Glass" ("Error Description"), s=w384, f=" - Rollo" ("Error Description")) -> (s? t:f=w394:string)
        n152 = Concatenate Strings(w394, " - Get Bootloader Seed and Key" ("Error Description")) -> (w390:string)
        n153 = call "EOL CAN_Get Bootloader Key.vi"("SA2 Operator"=w382, "Read Session in"=w380, "Write Session in"=w381) -> ("Response Good?"=w378:bool, "TxRx Data"=w379:string[][])  [unwired: 6 in, 1 out]
        n154 = And(x=w400, y=w378) -> (x .and. y?=w398:bool)
        n155 = Build Array (concatenate)(w386, w379) -> (w385:string[][])
        n156 = Not(x=w378) -> (.not. x?=w383:bool)
        n157 = case shown="False" w378 {
          tunnel: w396 -> [w402 w404]
          tunnel: [w403 w404] -> w395
          tunnel: w390 -> [w401 _]
          frame False {
            n158 = Concatenate Strings(w402, w401) -> (w403:string)
          }
          frame True {
          }
        }
        n159 = Bundle By Name(cluster=w399, "TxRx Data"=w385, "Response Good?"=w398, "Error String"=w395) -> (w397:T3)
        n160 = call "Insert Multiple Events.vi"("Insert all? (T)"=w383, "Events to Insert"=string[] ["Exit"], "Event queue in"=w388) -> ("Event queue out"=w389:string[])  [unwired: 4 in]
      }
      frame "Enable Production Mode" {
        n161 = Unbundle By Name(w425) -> ("Response Good?"=w426:bool, "TxRx Data"=w412:string[][], "Error String"=w422:string, "DSC Write Session in"=w408:refnum<k21>, "Read Session in"=w407:refnum<k21>, "Glass?"=w410:bool)
        n162 = Select(t=" - Glass" ("Error Description"), s=w410, f=" - Rollo" ("Error Description")) -> (s? t:f=w420:string)
        n163 = Concatenate Strings(w420, " - Enable Production Mode" ("Error Description")) -> (w416:string)
        n164 = call "EOL CAN_Enable_Production_Mode.vi"("Read Session in"=w407, "Write Session in"=w408) -> ("debug log"=w406:string[][], "Response Good?"=w405:bool)  [unwired: 7 in, 1 out]
        n165 = And(x=w426, y=w405) -> (x .and. y?=w424:bool)
        n166 = Build Array (concatenate)(w412, w406) -> (w411:string[][])
        n167 = Not(x=w405) -> (.not. x?=w409:bool)
        n168 = case shown="False" w405 {
          tunnel: w422 -> [w428 w430]
          tunnel: [w429 w430] -> w421
          tunnel: w416 -> [w427 _]
          frame False {
            n169 = Concatenate Strings(w428, w427) -> (w429:string)
          }
          frame True {
          }
        }
        n170 = Bundle By Name(cluster=w425, "TxRx Data"=w411, "Response Good?"=w424, "Error String"=w421) -> (w423:T3)
        n171 = call "Insert Multiple Events.vi"("Insert all? (T)"=w409, "Events to Insert"=string[] ["Exit"], "Event queue in"=w414) -> ("Event queue out"=w415:string[])  [unwired: 4 in]
      }
      frame "Disable Production Mode" {
        n172 = Unbundle By Name(w451) -> ("Response Good?"=w452:bool, "TxRx Data"=w438:string[][], "Error String"=w448:string, "DSC Write Session in"=w434:refnum<k21>, "Read Session in"=w433:refnum<k21>, "Glass?"=w436:bool)
        n173 = Select(t=" - Glass" ("Error Description"), s=w436, f=" - Rollo" ("Error Description")) -> (s? t:f=w446:string)
        n174 = Concatenate Strings(w446, " - Disable Production Mode" ("Error Description")) -> (w442:string)
        n175 = call "EOL CAN_Disable_Production_Mode.vi"("Read Session in"=w433, "Write Session in"=w434) -> ("debug log"=w432:string[][], "Response Good?"=w431:bool)  [unwired: 7 in, 1 out]
        n176 = And(x=w452, y=w431) -> (x .and. y?=w450:bool)
        n177 = Build Array (concatenate)(w438, w432) -> (w437:string[][])
        n178 = Not(x=w431) -> (.not. x?=w435:bool)
        n179 = case shown="False" w431 {
          tunnel: w448 -> [w454 w456]
          tunnel: [w455 w456] -> w447
          tunnel: w442 -> [w453 _]
          frame False {
            n180 = Concatenate Strings(w454, w453) -> (w455:string)
          }
          frame True {
          }
        }
        n181 = Bundle By Name(cluster=w451, "TxRx Data"=w437, "Response Good?"=w450, "Error String"=w447) -> (w449:T3)
        n182 = call "Insert Multiple Events.vi"("Insert all? (T)"=w435, "Events to Insert"=string[] ["Exit"], "Event queue in"=w440) -> ("Event queue out"=w441:string[])  [unwired: 4 in]
      }
      frame "Set Programming Date" {
        n183 = Unbundle By Name(w488) -> ("Response Good?"=w489:bool, "TxRx Data"=w475:string[][], "Error String"=w485:string, "DSC Write Session in"=w471:refnum<k21>, "Read Session in"=w470:refnum<k21>, "Glass?"=w473:bool)
        n184 = Format Date/Time String(time format string (%c)="%y,%m,%d") -> (date/time string=w458:string)  [unwired: 2 in]
        n185 = Spreadsheet String To Array(delimiter (Tab)=",", format string="%x", spreadsheet string=w458, array type (2D Dbl)=u8[] []) -> (array=w457:u8[])
        n186 = Select(t=" - Glass" ("Error Description"), s=w473, f=" - Rollo" ("Error Description")) -> (s? t:f=w483:string)
        n187 = Replace Array Subset(array=u8[] [6, 46, 241, 153, 85, 85, 85, 85] ("payload"), new element=w457, index=4) -> (w464:u8[])
        n188 = Concatenate Strings(w483, " - Set Program Date" ("Error Description")) -> (w479:string)
        n189 = Bundle By Name(cluster=T5 {"timestamp"=timestamp(0 s since 1904-01-01), "payload"=[6, 46, 241, 153, 85, 85, 85, 85], "identifier"=402391172, "type"=8, "extended?"=TRUE, "echo?"=FALSE} ("Tx CAN frame"), "payload"=w464) -> (w466:T5)
        n190 = call "EOL CAN_Send_Single_Message.vi"("Tx CAN frame"=w466, "Read Session in"=w470, "Write Session in"=w471) -> ("Response Good?"=w468:bool, "TxRx Data"=w469:string[][])  [unwired: 4 in, 3 out]
        n191 = And(x=w489, y=w468) -> (x .and. y?=w487:bool)
        n192 = Build Array (concatenate)(w475, w469) -> (w474:string[][])
        n193 = Not(x=w468) -> (.not. x?=w472:bool)
        n194 = case shown="False" w468 {
          tunnel: w485 -> [w491 w493]
          tunnel: [w492 w493] -> w484
          tunnel: w479 -> [w490 _]
          frame False {
            n195 = Concatenate Strings(w491, w490) -> (w492:string)
          }
          frame True {
          }
        }
        n196 = Bundle By Name(cluster=w488, "TxRx Data"=w474, "Response Good?"=w487, "Error String"=w484) -> (w486:T3)
        n197 = call "Insert Multiple Events.vi"("Insert all? (T)"=w472, "Events to Insert"=string[] ["Exit"], "Event queue in"=w477) -> ("Event queue out"=w478:string[])  [unwired: 4 in]
      }
      frame "Set Start Routine 2" {
        n198 = Unbundle By Name(w518) -> ("Response Good?"=w519:bool, "TxRx Data"=w505:string[][], "Error String"=w515:string, "DSC Write Session in"=w501:refnum<k21>, "Read Session in"=w500:refnum<k21>, "Glass?"=w503:bool)
        n199 = flat-sequence {
          tunnel: [errorcluster {"status"=FALSE, "code"=0, "source"=""} ("Error in")] -> w494
          frame #0 {
            n200 = Wait (ms)(milliseconds to wait=u32 10) -> ()  [unwired: 1 out]
          }
        }
        n201 = Select(t=" - Glass" ("Error Description"), s=w503, f=" - Rollo" ("Error Description")) -> (s? t:f=w513:string)
        n202 = Concatenate Strings(w513, " - Set Program Date" ("Error Description")) -> (w509:string)
        n203 = call "EOL CAN_Send_Single_Message.vi"("Retries"=10, "Msg Wait Time"=u32 400, "Error in"=w494, "Tx CAN frame"=T5 {"timestamp"=timestamp(0 s since 1904-01-01), "payload"=[7, 49, 1, 255, 0, 2, 113, 0], "identifier"=402391172, "type"=8, "extended?"=TRUE, "echo?"=FALSE}, "Read Session in"=w500, "Write Session in"=w501) -> ("Response Good?"=w498:bool, "TxRx Data"=w499:string[][])  [unwired: 1 in, 3 out]
        n204 = And(x=w519, y=w498) -> (x .and. y?=w517:bool)
        n205 = Build Array (concatenate)(w505, w499) -> (w504:string[][])
        n206 = Not(x=w498) -> (.not. x?=w502:bool)
        n207 = case shown="False" w498 {
          tunnel: w515 -> [w523 w525]
          tunnel: [w524 w525] -> w514
          tunnel: w509 -> [w522 _]
          frame False {
            n208 = Concatenate Strings(w523, w522) -> (w524:string)
          }
          frame True {
          }
        }
        n209 = Bundle By Name(cluster=w518, "TxRx Data"=w504, "Response Good?"=w517, "Error String"=w514) -> (w516:T3)
        n210 = call "Insert Multiple Events.vi"("Insert all? (T)"=w502, "Events to Insert"=string[] ["Exit"], "Event queue in"=w507) -> ("Event queue out"=w508:string[])  [unwired: 4 in]
      }
      frame "Set Blah 2" {
        n211 = Unbundle By Name(w549) -> ("Response Good?"=w550:bool, "TxRx Data"=w536:string[][], "Error String"=w546:string, "DSC Write Session in"=w532:refnum<k21>, "Read Session in"=w531:refnum<k21>, "Glass?"=w534:bool)
        n212 = Select(t=" - Glass" ("Error Description"), s=w534, f=" - Rollo" ("Error Description")) -> (s? t:f=w544:string)
        n213 = Concatenate Strings(w544, " - Set Program Date" ("Error Description")) -> (w540:string)
        n214 = call "EOL CAN_Send_Single_Message.vi"("Retries"=10, "Msg Wait Time"=u32 100, "Tx CAN frame"=T5 {"timestamp"=timestamp(0 s since 1904-01-01), "payload"=[7, 46, 241, 161, 48, 48, 48, 48], "identifier"=402391172, "type"=8, "extended?"=TRUE, "echo?"=FALSE}, "Read Session in"=w531, "Write Session in"=w532) -> ("Response Good?"=w526:bool, "TxRx Data"=w530:string[][])  [unwired: 2 in, 3 out]
        n215 = And(x=w550, y=w526) -> (x .and. y?=w548:bool)
        n216 = Build Array (concatenate)(w536, w530) -> (w535:string[][])
        n217 = Not(x=w526) -> (.not. x?=w533:bool)
        n218 = case shown="False" w526 {
          tunnel: w546 -> [w552 w554]
          tunnel: [w553 w554] -> w545
          tunnel: w540 -> [w551 _]
          frame False {
            n219 = Concatenate Strings(w552, w551) -> (w553:string)
          }
          frame True {
          }
        }
        n220 = Bundle By Name(cluster=w549, "TxRx Data"=w535, "Response Good?"=w548, "Error String"=w545) -> (w547:T3)
        n221 = call "Insert Multiple Events.vi"("Insert all? (T)"=w533, "Events to Insert"=string[] ["Exit"], "Event queue in"=w538) -> ("Event queue out"=w539:string[])  [unwired: 4 in]
      }
      frame "Set Blah 3" {
        w555 = TRUE ("y")
        n222 = Unbundle By Name(w578) -> ("Response Good?"=w579:bool, "TxRx Data"=w565:string[][], "Error String"=w575:string, "DSC Write Session in"=w561:refnum<k21>, "Read Session in"=w560:refnum<k21>, "Glass?"=w563:bool)
        n223 = Select(t=" - Glass" ("Error Description"), s=w563, f=" - Rollo" ("Error Description")) -> (s? t:f=w573:string)
        n224 = Concatenate Strings(w573, " - Set Program Date" ("Error Description")) -> (w569:string)
        n225 = call "EOL CAN_Send_Single_Message.vi"("Retries"=10, "Msg Wait Time"=u32 100, "Tx CAN frame"=T5 {"timestamp"=timestamp(0 s since 1904-01-01), "payload"=[3, 40, 1, 1, 85, 85, 85, 85], "identifier"=402391172, "type"=8, "extended?"=TRUE, "echo?"=FALSE}, "Read Session in"=w560, "Write Session in"=w561) -> ("TxRx Data"=w559:string[][])  [unwired: 2 in, 4 out]
        n226 = And(x=w579, y=w555) -> (x .and. y?=w577:bool)
        n227 = Build Array (concatenate)(w565, w559) -> (w564:string[][])
        n228 = Not(x=w555) -> (.not. x?=w562:bool)
        n229 = case shown="False" w555 {
          tunnel: w575 -> [w581 w583]
          tunnel: [w582 w583] -> w574
          tunnel: w569 -> [w580 _]
          frame False {
            n230 = Concatenate Strings(w581, w580) -> (w582:string)
          }
          frame True {
          }
        }
        n231 = Bundle By Name(cluster=w578, "TxRx Data"=w564, "Response Good?"=w577, "Error String"=w574) -> (w576:T3)
        n232 = call "Insert Multiple Events.vi"("Insert all? (T)"=w562, "Events to Insert"=string[] ["Exit"], "Event queue in"=w567) -> ("Event queue out"=w568:string[])  [unwired: 4 in]
      }
      frame "Set Start Routine 1" {
        w584 = TRUE
        n233 = Unbundle By Name(w605) -> ("Response Good?"=w606:bool, "TxRx Data"=w592:string[][], "Error String"=w602:string, "DSC Write Session in"=w588:refnum<k21>, "Read Session in"=w587:refnum<k21>, "Glass?"=w590:bool)
        n234 = Select(t=" - Glass" ("Error Description"), s=w590, f=" - Rollo" ("Error Description")) -> (s? t:f=w600:string)
        n235 = Concatenate Strings(w600, " - Set Program Date" ("Error Description")) -> (w596:string)
        n236 = call "EOL CAN_Send_Single_Message.vi"("Tx CAN frame"=T5 {"timestamp"=timestamp(0 s since 1904-01-01), "payload"=[4, 49, 1, 2, 3, 85, 85, 85], "identifier"=402391172, "type"=8, "extended?"=TRUE, "echo?"=FALSE}, "Read Session in"=w587, "Write Session in"=w588) -> ("TxRx Data"=w586:string[][])  [unwired: 4 in, 4 out]
        n237 = And(x=w606, y=w584) -> (x .and. y?=w604:bool)
        n238 = Build Array (concatenate)(w592, w586) -> (w591:string[][])
        n239 = Not(x=w584) -> (.not. x?=w589:bool)
        n240 = case shown="False" w584 {
          tunnel: w602 -> [w608 w610]
          tunnel: [w609 w610] -> w601
          tunnel: w596 -> [w607 _]
          frame False {
            n241 = Concatenate Strings(w608, w607) -> (w609:string)
          }
          frame True {
          }
        }
        n242 = Bundle By Name(cluster=w605, "TxRx Data"=w591, "Response Good?"=w604, "Error String"=w601) -> (w603:T3)
        n243 = call "Insert Multiple Events.vi"("Insert all? (T)"=w589, "Events to Insert"=string[] ["Exit"], "Event queue in"=w594) -> ("Event queue out"=w595:string[])  [unwired: 4 in]
      }
      frame "Activate Development Frames" {
        n244 = Unbundle By Name(w632) -> ("Response Good?"=w633:bool, "TxRx Data"=w619:string[][], "Error String"=w629:string, "DSC Write Session in"=w615:refnum<k21>, "Read Session in"=w614:refnum<k21>, "Glass?"=w617:bool)
        n245 = Select(t=" - Glass" ("Error Description"), s=w617, f=" - Rollo" ("Error Description")) -> (s? t:f=w627:string)
        n246 = Concatenate Strings(w627, " - Activate Dev Frames" ("Error Description")) -> (w623:string)
        n247 = call "EOL CAN_Send_Single_Message.vi"("Tx CAN frame"=T5 {"timestamp"=timestamp(0 s since 1904-01-01), "payload"=[4, 46, 9, 2, 128, 85, 85, 85], "identifier"=402391172, "type"=8, "extended?"=TRUE, "echo?"=FALSE}, "Read Session in"=w614, "Write Session in"=w615) -> ("Response Good?"=w612:bool, "TxRx Data"=w613:string[][])  [unwired: 4 in, 3 out]
        n248 = And(x=w633, y=w612) -> (x .and. y?=w631:bool)
        n249 = Build Array (concatenate)(w619, w613) -> (w618:string[][])
        n250 = Not(x=w612) -> (.not. x?=w616:bool)
        n251 = case shown="False" w612 {
          tunnel: w629 -> [w635 w637]
          tunnel: [w636 w637] -> w628
          tunnel: w623 -> [w634 _]
          frame False {
            n252 = Concatenate Strings(w635, w634) -> (w636:string)
          }
          frame True {
          }
        }
        n253 = Bundle By Name(cluster=w632, "TxRx Data"=w618, "Response Good?"=w631, "Error String"=w628) -> (w630:T3)
        n254 = call "Insert Multiple Events.vi"("Insert all? (T)"=w616, "Events to Insert"=string[] ["Exit"], "Event queue in"=w621) -> ("Event queue out"=w622:string[])  [unwired: 4 in]
      }
      frame "Set Key Off On Reset" {
        n255 = Unbundle By Name(w659) -> ("Response Good?"=w660:bool, "TxRx Data"=w646:string[][], "Error String"=w656:string, "DSC Write Session in"=w642:refnum<k21>, "Read Session in"=w641:refnum<k21>, "Glass?"=w644:bool)
        n256 = Select(t=" - Glass" ("Error Description"), s=w644, f=" - Rollo" ("Error Description")) -> (s? t:f=w654:string)
        n257 = Concatenate Strings(w654, " - Key Off On Reset" ("Error Description")) -> (w650:string)
        n258 = call "EOL CAN_Send_Single_Message.vi"("Tx CAN frame"=T5 {"timestamp"=timestamp(0 s since 1904-01-01), "payload"=[2, 17, 2, 85, 85, 85, 85, 85], "identifier"=402391172, "type"=8, "extended?"=TRUE, "echo?"=FALSE}, "Read Session in"=w641, "Write Session in"=w642) -> ("Response Good?"=w639:bool, "TxRx Data"=w640:string[][])  [unwired: 4 in, 3 out]
        n259 = And(x=w660, y=w639) -> (x .and. y?=w658:bool)
        n260 = Build Array (concatenate)(w646, w640) -> (w645:string[][])
        n261 = Not(x=w639) -> (.not. x?=w643:bool)
        n262 = case shown="False" w639 {
          tunnel: w656 -> [w662 w664]
          tunnel: [w663 w664] -> w655
          tunnel: w650 -> [w661 _]
          frame False {
            n263 = Concatenate Strings(w662, w661) -> (w663:string)
          }
          frame True {
          }
        }
        n264 = Bundle By Name(cluster=w659, "TxRx Data"=w645, "Response Good?"=w658, "Error String"=w655) -> (w657:T3)
        n265 = call "Insert Multiple Events.vi"("Insert all? (T)"=w643, "Events to Insert"=string[] ["Exit"], "Event queue in"=w648) -> ("Event queue out"=w649:string[])  [unwired: 4 in]
      }
      frame "Clear DTC" {
        n266 = Unbundle By Name(w685) -> ("Response Good?"=w686:bool, "TxRx Data"=w672:string[][], "Error String"=w682:string, "DSC Write Session in"=w668:refnum<k21>, "Read Session in"=w667:refnum<k21>, "Glass?"=w670:bool)
        n267 = Select(t=" - Glass" ("Error Description"), s=w670, f=" - Rollo" ("Error Description")) -> (s? t:f=w680:string)
        n268 = Concatenate Strings(w680, " - Clear DTC" ("Error Description")) -> (w676:string)
        n269 = call "EOL CAN_Clear_DTC's.vi"("Read Session in"=w667, "Write Session in"=w668) -> ("TxRx Data"=w666:string[][], "Response Good?"=w665:bool)  [unwired: 7 in, 1 out]
        n270 = And(x=w686, y=w665) -> (x .and. y?=w684:bool)
        n271 = Build Array (concatenate)(w672, w666) -> (w671:string[][])
        n272 = Not(x=w665) -> (.not. x?=w669:bool)
        n273 = case shown="False" w665 {
          tunnel: w682 -> [w688 w690]
          tunnel: [w689 w690] -> w681
          tunnel: w676 -> [w687 _]
          frame False {
            n274 = Concatenate Strings(w688, w687) -> (w689:string)
          }
          frame True {
          }
        }
        n275 = Bundle By Name(cluster=w685, "TxRx Data"=w671, "Response Good?"=w684, "Error String"=w681) -> (w683:T3)
        n276 = call "Insert Multiple Events.vi"("Insert all? (T)"=w669, "Events to Insert"=string[] ["Exit"], "Event queue in"=w674) -> ("Event queue out"=w675:string[])  [unwired: 4 in]
      }
      frame "Exit" {
        n277 = Unbundle By Name(w694) -> ("Response Good?"=→"Response Good?":bool, "Error String"=→"Error String Out":string, "TxRx Data"=→"TxRx Data":string[][])
      }
    }
  }
